vi "Sensor FGV.vi"(7 "Enum":T1, 8 "error in (no error)":errorcluster, 10 "Boolean in":bool) -> (0 "error out":errorcluster, 2 "Boolean out":bool)   [LabVIEW 2013]
uses:
  Controls/Sensor.ctl
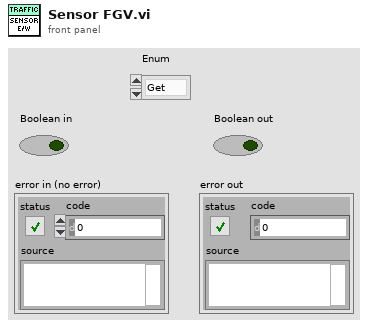
[diagram p1: front panel]
types:
  T1 = typedef "Sensor.ctl" = enum16{"Get", "Set"}
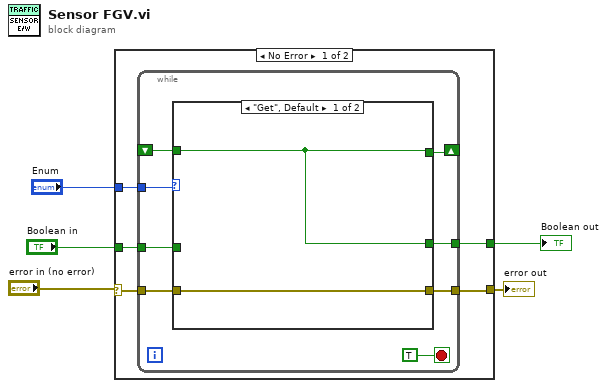
[diagram p0: block diagram]
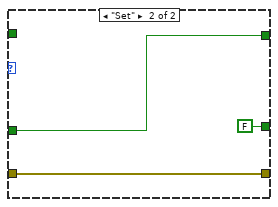
[diagram p2: hidden frame]
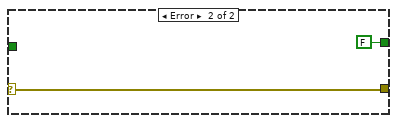
[diagram p3: hidden frame]
diagram:
  n1 = case shown="No Error" "error in (no error)" {
    selector: "error in (no error)" -> [w6 w25]
    tunnel: "Enum" -> [w10 _]
    tunnel: "Boolean in" -> [w9 _]
    tunnel: [w8 FALSE ("Boolean")] -> w3
    tunnel: [w7 w25] -> w5
    frame No Error {
      n2 = while {
        tunnel: w10 -> [w18]
        tunnel: w9 -> [w17]
        shift-right: [w16] -> _
        shift-left: _ -> [w15]
        tunnel: [w14] -> w8
        tunnel: [w13] -> w7
        tunnel: w6 -> [w12]
        stop <- TRUE stop-if-true
        n3 = case shown="\"Get\", Default" w18 {
          tunnel: w17 -> [_ w23]
          tunnel: [w20 w23] -> w16
          tunnel: w15 -> [w20 _]
          tunnel: [w20 FALSE ("Boolean")] -> w14
          tunnel: [w19 w21] -> w13
          tunnel: w12 -> [w19 w21]
          frame "Get", Default {
          }
          frame "Set" {
          }
        }
      }
    }
    frame Error {
    }
  }
  "error out" <- w5
  "Boolean out" <- w3
